vi "3D_Position_Graph.vi"() -> ()   [LabVIEW 2018]
uses:
  <vilib>/Native 3D Graph/xcontrol/3DPC_SurfacePlot.xctl
panel:
  out "3D Graph":refnum<class "Base Datatype.lvclass">[](xcontrol)
  in  "velocity":dbl
  out "zPosition":dbl
  out "xPosition":dbl
  out "vZfinal":dbl
  out "vXfinal":dbl
  out "vZinitial":dbl
  out "vXinitial":dbl
  out "yPosition":dbl
  out "vYfinal":dbl
  out "timeOfFlight":dbl format="%#_5g"
  in  "bField":dbl
  in  "height":dbl
  out "vYinitial":dbl
  in  "eField":dbl
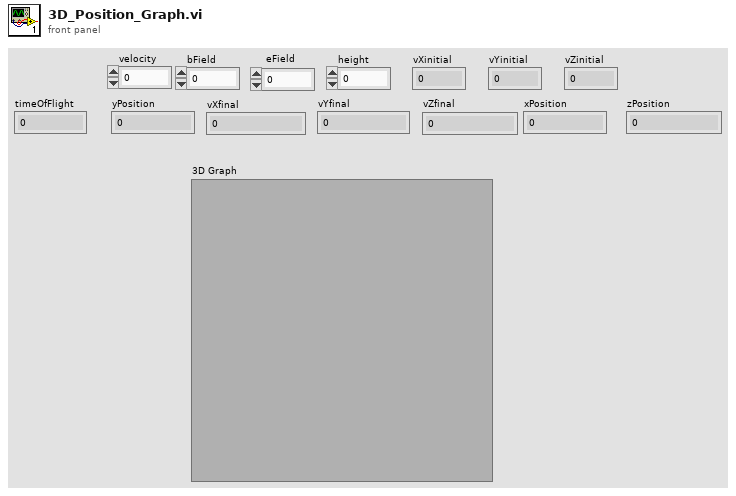
[diagram p1: front panel]
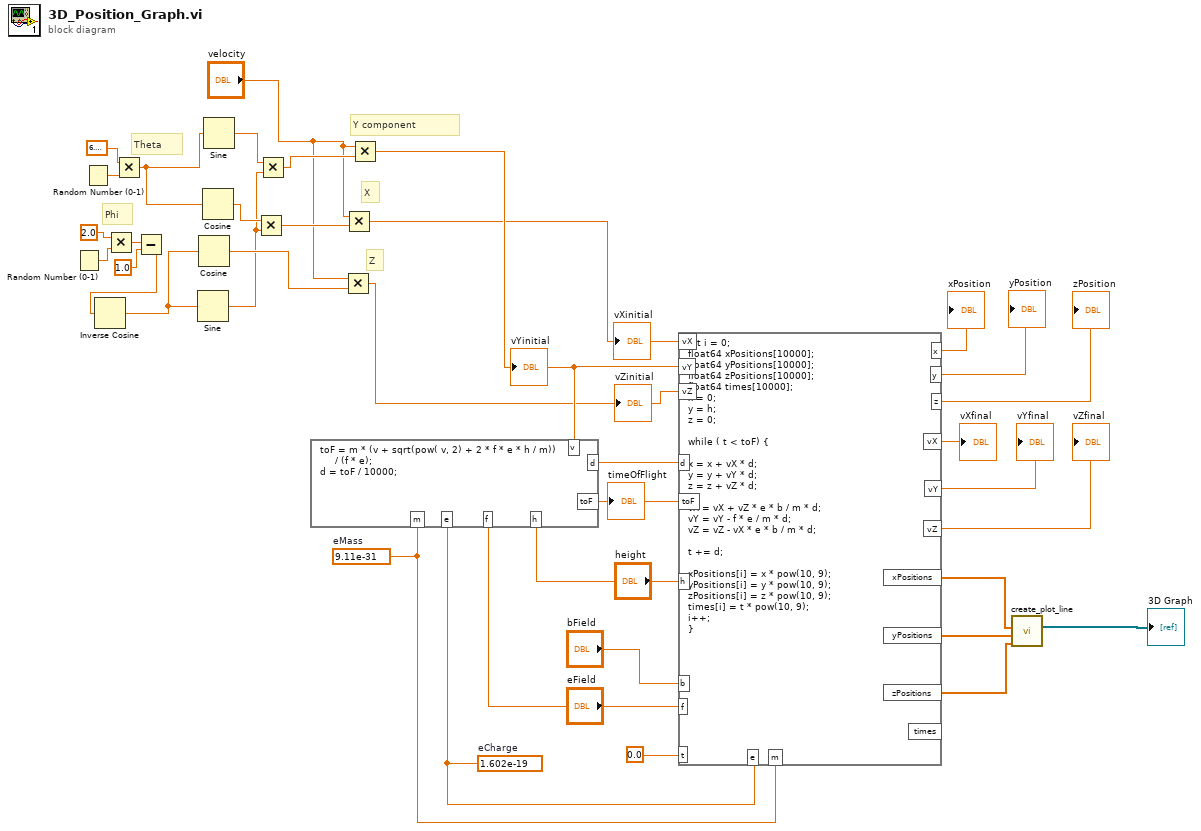
[diagram p0: block diagram]
diagram:
  w35 = 1.602e-19  # eCharge
  w34 = 9.11e-31  # eMass
  # "Phi"
  # "Theta"
  # "Z"
  # "X"
  # "Y component"
  n1 = Random Number (0-1)() -> (number: 0 to 1=w17:dbl)
  n2 = Random Number (0-1)() -> (number: 0 to 1=w20:dbl)
  n3 = Multiply(x=2.0, y=w17) -> (x*y=w16:dbl)
  n4 = Multiply(x=6.283185307179586, y=w20) -> (x*y=w14:dbl)
  n5 = Subtract(x=w16, y=1.0) -> (x-y=w13:dbl)
  n6 = Inverse Cosine(1:w13) -> (0:w12:dbl)
  n7 = Sine(x=w12) -> (sin(x)=w7:dbl)
  n8 = Cosine(x=w12) -> (cos(x)=w11:dbl)
  n9 = Cosine(x=w14) -> (cos(x)=w8:dbl)
  n10 = Sine(x=w14) -> (sin(x)=w10:dbl)
  n11 = Multiply(x=w8, y=w7) -> (x*y=w6:dbl)
  n12 = Multiply(x=w10, y=w7) -> (x*y=w9:dbl)
  n13 = Multiply(x="velocity", y=w11) -> (x*y=w3:dbl)
  "vZinitial" <- w3
  n14 = Multiply(x="velocity", y=w6) -> (x*y=w4:dbl)
  "vXinitial" <- w4
  n15 = Multiply(x="velocity", y=w9) -> (x*y=w5:dbl)
  "vYinitial" <- w5
  n16 = formula code="toF = m * (v + sqrt(pow( v, 2) + 2 * f * e * h / m))\n     / (f * e);\nd = toF / 10000;"("f"="eField", "h"="height", "v"=w5, "m"=w34, "e"=w35) -> ("toF"=w32:dbl, "d"=w33:dbl)
  "timeOfFlight" <- w32
  n17 = formula code="int i = 0;\nfloat64 xPositions[10000];\nfloat64 yPositions[10000];\nfloat64 zPositions[10000];\nfloat64 times[10000];\nx = 0;\ny = h;\nz = 0;\n\nwhile ( t < toF) {\n\nx = x + vX * d;\ny = y + vY * d;\nz = z + vZ * d;\n\nvX = vX + vZ * e * b / m * d;\nvY = vY - f * e / m * d;\nvZ = vZ - vX * e * b / m * d;\n\nt += d;\n\nxPositions[i] = x * pow(10, 9);\nyPositions[i] = y * pow(10, 9);\nzPositions[i] = z * pow(10, 9);\ntimes[i] = t * pow(10, 9);\ni++;\n}"("vY"=w5, "e"=w35, "m"=w34, "f"="eField", "d"=w33, "h"="height", "toF"=w32, "t"=0.0, "b"="bField", "vX"=w4, "vZ"=w3) -> ("y"=→"yPosition":dbl, "vY"=→"vYfinal":dbl, "vX"=→"vXfinal":dbl, "vZ"=→"vZfinal":dbl, "x"=→"xPosition":dbl, "z"=→"zPosition":dbl, "xPositions"=w23:dbl[], "yPositions"=w22:dbl[], "zPositions"=w21:dbl[])  [unwired: 1 out]
  n18 = call <vilib>:"create_plot_line.vi"("z vector"=w21, "y vector"=w22, "x vector"=w23) -> ("plots out"=→"3D Graph":refnum<class "Base Datatype.lvclass">[])  [unwired: 2 in, 6 out]
